vi "Get All Available GU.vi"(8 "error in":errorcluster, 10 "GU Bench File Path":path) -> (0 "error out":errorcluster, 2 "GU Numbers Out":i32[](array[numeric]))   [LabVIEW 2020, in "GUCalibration2.lvlib"]
uses:
  GUCalibration2.lvlib
  Controls/Error Enum.ctl
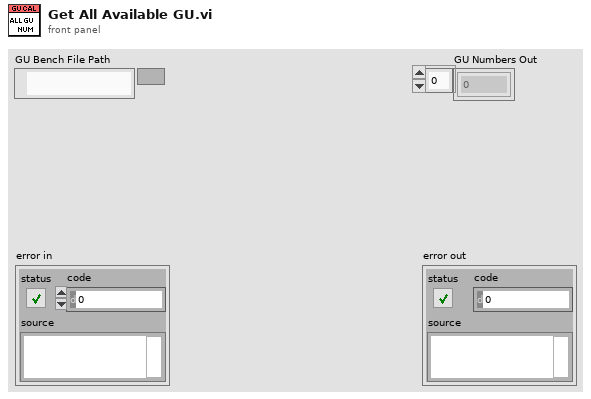
[diagram p1: front panel]
types:
  T1 = typedef "GUCalibration2.lvlib/Error Enum.ctl" = enum16{"Error Template Case", "Duplicated GU Number", "Test Items Mismatch"}
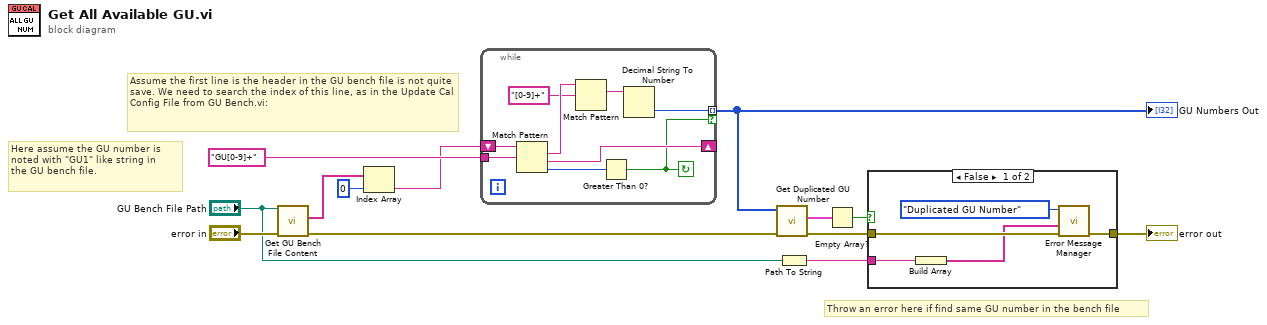
[diagram p0: block diagram]
diagram:
  # "Throw an error here if find same GU number in the bench file"
  # "Here assume the GU number is noted with \"GU1\" like string in\nthe GU bench file."
  # "Assume the first line is the header in the GU bench file is not quite save. We need to search the index of this line, as in the Update Cal Config File from GU Bench.vi:"
  n1 = call "Get GU Bench File Content.vi"("error in"="error in", "GU Bench File Path"="GU Bench File Path") -> ("error out"=w7:errorcluster, "Get GU Bench Content"=w5:string[])  [unwired: 8 in]
  n2 = Index Array(array=w5, index=0 ("index (row)")) -> (element=w11:string)
  n3 = while {
    tunnel: "GU[0-9]+" ("GU Name Format") -> [w21]
    shift-right: [w20] -> _
    shift-left: w11 -> [w22]
    tunnel: [w14] -> w10 mode=indexing if=w18
    stop <- w18 continue-if-true
    n4 = Match Pattern(string=w22, regular expression=w21) -> (match substring=w17:string, after substring=w20:string, offset past match=w19:i32)  [unwired: 1 in, 1 out]
    n5 = Match Pattern(string=w17, regular expression="[0-9]+") -> (match substring=w15:string)  [unwired: 1 in, 3 out]
    n6 = Greater Than 0?(x=w19) -> (x > 0?=w18:bool)
    n7 = Decimal String To Number(string=w15) -> (number=w14:i32)  [unwired: 2 in, 1 out]
  }
  "GU Numbers Out" <- w10
  n8 = call "Get Duplicated GU Number.vi"("error in"=w7, "GU Numbers"=w10) -> ("error out"=w4:errorcluster, "Repeated GU"=w9:cluster{"GU Number":i32, "Index":i32[]}[])  [unwired: 8 in]
  n9 = Path To String(path="GU Bench File Path") -> (string=w1:string)
  n10 = Empty Array?(array=w9) -> (empty?=w2:bool)
  n11 = case shown="False" w2 {
    tunnel: w4 -> [w27 w28]
    tunnel: [w26 w28] -> w3
    tunnel: w1 -> [w24 _]
    frame False {
      n12 = Build Array(w24) -> (w23:string[])
      n13 = call "Error Message Manager.vi"("error in"=w27, "Variable Msg"=w23, "Error Selection"=Error_Enum."Duplicated GU Number") -> ("error out"=w26:errorcluster)  [unwired: 8 in]
    }
    frame True {
    }
  }
  "error out" <- w3
